vi "LS372_set_Monitor_Values.vi"(4 "LS372-Status":T1, 5 "System Monitor Variables (in)":T2) -> (1 "System Monitor Variables (out)":T2)   [LabVIEW 2019]
uses:
  Global/Global Variables/System Monitor Cluster.ctl
  LS372/LS372-Status.ctl
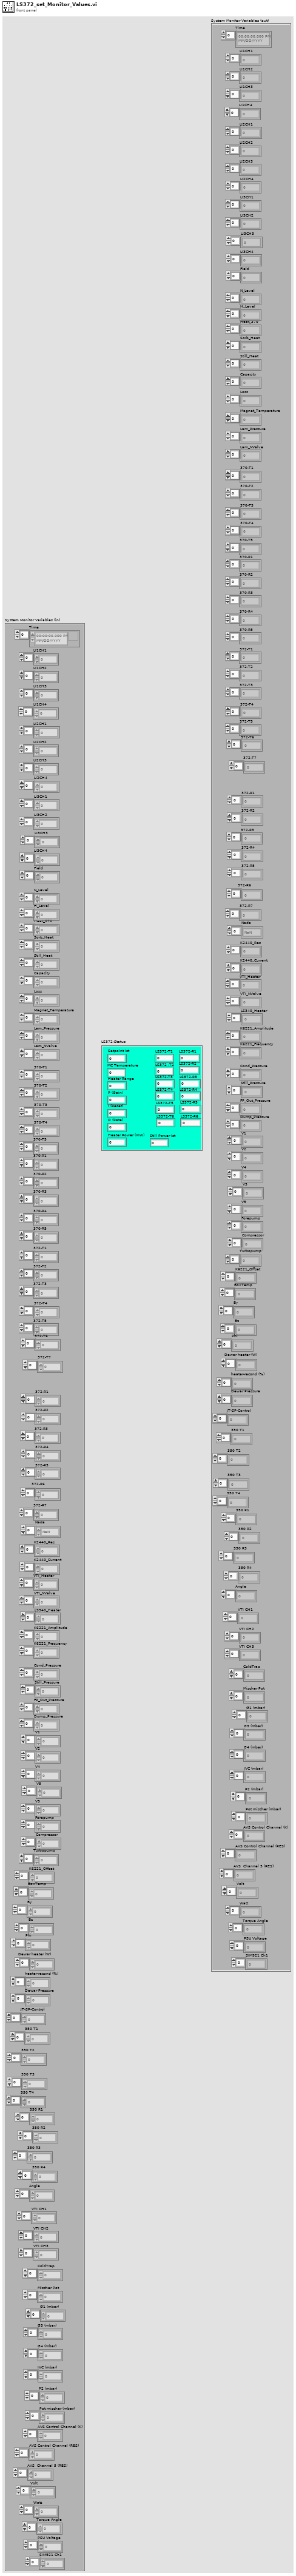
[diagram p1: front panel]
types:
  T1 = typedef "LS372-Status.ctl" = cluster{"Heater Range":dbl, "P (Gain)":dbl, "I (Reset)":dbl, "D (Rate)":dbl, "Heater Power (mW)":dbl, "MC Temperature":dbl, "LS372-T1":dbl, "LS372 -T2":dbl, "LS372-R1 ":dbl, "LS372-R2":dbl, "LS372-T3":dbl, "LS372-T4":dbl, "LS372-R3 ":dbl, "LS372-R4 \n\n\n\n":dbl, "LS372-T5":dbl, "LS372-T6":dbl, "LS372-R5":dbl, "LS372-R6 ":dbl, "Still Power ist":dbl, "Setpoint ist":dbl}
  T2 = typedef "System Monitor Cluster.ctl" = cluster{"Time":timestamp[], "LI1CH1":dbl[], "LI1CH2":dbl[], "LI2CH1":dbl[], "LI2CH2":dbl[], "LI3CH1":dbl[], "LI3CH2":dbl[], "Field":dbl[], "N_Level":dbl[], "H_Level":dbl[], "Heat_370":dbl[], "Sorb_Heat":dbl[], "Still_Heat":dbl[], "Capacity":dbl[], "Loss":dbl[], "Magnet_Temperature":dbl[], "Lam_Pressure":dbl[], "Lam_NValve":dbl[], "370-T1":dbl[], "370-T2":dbl[], "370-T3":dbl[], "370-T4":dbl[], "370-T5":dbl[], "370-R1":dbl[], "370-R2":dbl[], "370-R3":dbl[], "370-R4":dbl[], "370-R5":dbl[], "372-T1":dbl[], "372-T2":dbl[], "372-T3":dbl[], "372-T4":dbl[], "372-T5":dbl[], "372-T6":dbl[], "372-R1":dbl[], "372-R2":dbl[], "372-R3":dbl[], "372-R4":dbl[], "372-R5":dbl[], "372-R6":dbl[], "Nada":dbl[], "K2440_Res":dbl[], "K2440_Current":dbl[], "VTI_Heater":dbl[], "VTI_NValve":dbl[], "LS340_Heater":dbl[], "K6221_Amplitude":dbl[], "K6221_Frequency":dbl[], "Cond_Pressure":dbl[], "Still_Pressure":dbl[], "FP_Out_Pressure":dbl[], "Dump_Pressure":dbl[], "V1":dbl[], "V2":dbl[], "V4":dbl[], "V5":dbl[], "V9":dbl[], "Forepump":dbl[], "Compressor":dbl[], "K6221_Offset":dbl[], "BoxTemp":dbl[], "By":dbl[], "Bz":dbl[], "Phi":dbl[], "heater-recond (%)":dbl[], "Dewar Pressure ":dbl[], "JT-SP-Control":dbl[], "350 T1":dbl[], "350 T2":dbl[], "350 T3":dbl[], "350 T4":dbl[], "350 R1":dbl[], "350 R2":dbl[], "350 R3":dbl[], "350 R4":dbl[], "Angle":dbl[], "VTI CH1":dbl[], "VTI CH2":dbl[], "VTI CH3":dbl[], "ColdTrap":dbl[], "Mischer Pot":dbl[], "G1 (mbar)":dbl[], "G3 (mbar) ":dbl[], "G4 (mbar)":dbl[], "IVC (mbar)":dbl[], "P2 (mbar) ":dbl[], "Pot mischer (mbar)":dbl[], "AVS Control Channel (K)":dbl[], "AVS Control Channel (RES)":dbl[], "AVS  Channel 5 (RES) ":dbl[], "LI3CH3":dbl[], "LI3CH4":dbl[], "LI1CH3":dbl[], "LI1CH4":dbl[], "LI2CH3":dbl[], "LI2CH4":dbl[], "Volt":dbl[], "Watt":dbl[], "Torque Angle":dbl[], "Dewar heater (W)":dbl[], "PSU Voltage":dbl[], "Turbopump":dbl[], "372-R7":dbl[], "372-T7":dbl[], "SIM921 Ch1":dbl[]}
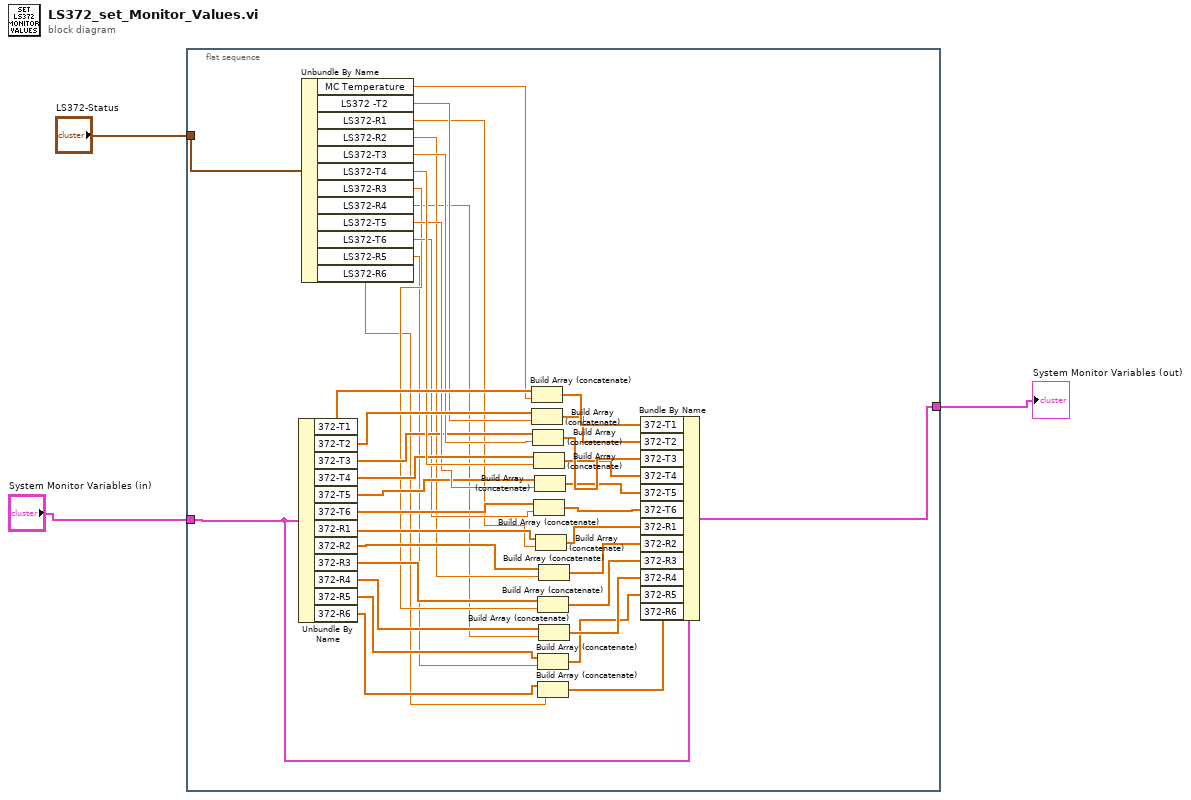
[diagram p0: block diagram]
diagram:
  n1 = flat-sequence {
    tunnel: "LS372-Status" -> [w42]
    tunnel: [w40] -> w2
    tunnel: "System Monitor Variables (in)" -> [w41]
    frame #0 {
      n2 = Unbundle By Name(w41) -> ("372-T1"=w27:dbl[], "372-T2"=w25:dbl[], "372-T3"=w18:dbl[], "372-T4"=w22:dbl[], "372-T5"=w20:dbl[], "372-T6"=w17:dbl[], "372-R1"=w15:dbl[], "372-R2"=w13:dbl[], "372-R3"=w11:dbl[], "372-R4"=w9:dbl[], "372-R5"=w7:dbl[], "372-R6"=w5:dbl[])
      n3 = Unbundle By Name(w42) -> ("MC Temperature"=w26:dbl, "LS372 -T2"=w24:dbl, "LS372-R1"=w14:dbl, "LS372-R2"=w12:dbl, "LS372-T3"=w19:dbl, "LS372-T4"=w23:dbl, "LS372-R3"=w10:dbl, "LS372-R4"=w8:dbl, "LS372-T5"=w21:dbl, "LS372-T6"=w16:dbl, "LS372-R5"=w6:dbl, "LS372-R6"=w4:dbl)
      n4 = Build Array (concatenate)(w27, w26) -> (w39:dbl[])
      n5 = Build Array (concatenate)(w25, w24) -> (w38:dbl[])
      n6 = Build Array (concatenate)(w18, w19) -> (w37:dbl[])
      n7 = Build Array (concatenate)(w22, w23) -> (w36:dbl[])
      n8 = Build Array (concatenate)(w17, w16) -> (w34:dbl[])
      n9 = Build Array (concatenate)(w20, w21) -> (w35:dbl[])
      n10 = Build Array (concatenate)(w15, w14) -> (w33:dbl[])
      n11 = Build Array (concatenate)(w11, w10) -> (w31:dbl[])
      n12 = Build Array (concatenate)(w7, w6) -> (w29:dbl[])
      n13 = Build Array (concatenate)(w5, w4) -> (w28:dbl[])
      n14 = Build Array (concatenate)(w13, w12) -> (w32:dbl[])
      n15 = Build Array (concatenate)(w9, w8) -> (w30:dbl[])
      n16 = Bundle By Name(cluster=w41, "372-T1"=w39, "372-T2"=w38, "372-T3"=w37, "372-T4"=w36, "372-T5"=w35, "372-T6"=w34, "372-R1"=w33, "372-R2"=w32, "372-R3"=w31, "372-R4"=w30, "372-R5"=w29, "372-R6"=w28) -> (w40:T2)
    }
  }
  "System Monitor Variables (out)" <- w2
